vi "configure.vi"(8 "error in (no error)":errorcluster, 11 "lv-build-default in":refnum<class "lv-builder.lvclass">) -> (0 "error out":errorcluster, 3 "lv-build-default out":refnum<class "lv-builder.lvclass">)   [LabVIEW 2015, in "lv-builder.lvlib" / "lv-builder.lvclass"]
uses:
  lv-builder.lvclass
  lv-builder.lvclass/lv-builder.ctl
  private/_controls/command_configuration.ctl
  lv-builder.lvlib
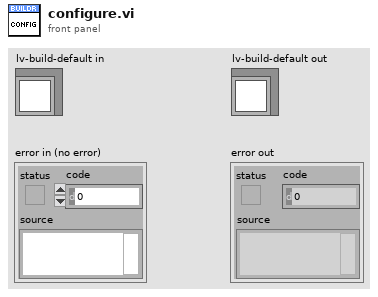
[diagram p1: front panel]
types:
  T1 = typedef "lv-builder.lvlib/command_configuration.ctl" = enum16{"<config_command>", "read_config", "write_config", "<null>"}
  T2 = typedef "lv-builder.lvlib/configuration.ctl" = cluster{"lvlibp_directory":string, "zip_directory":string, "lvlib_directory":string, "update_version_vi":string, "installer_post_file":string, "lvlib_post_action":u16, "installer_post_action":u16, "application_post_action":u16, "zip_post_action":u16}
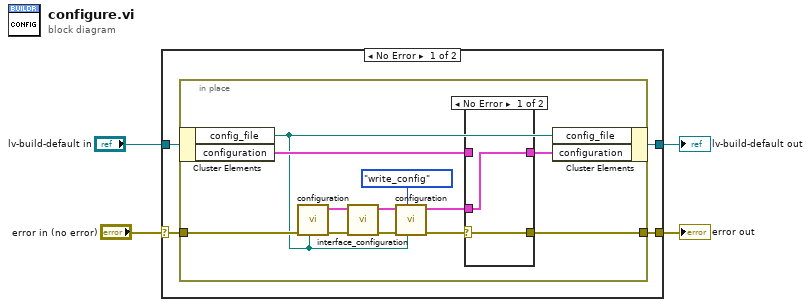
[diagram p0: block diagram]
diagram:
  n1 = case shown="No Error" "error in (no error)" {
    selector: "error in (no error)" -> [w8 w26]
    tunnel: "lv-build-default in" -> [w6 w25]
    tunnel: [w7 w26] -> w2
    tunnel: [w5 w25] -> w1
    frame No Error {
      n2 = in-place {
        in-place-border: w8 -> [w13]
        in-place-border: [w20] -> w7
        n3 = in-place-cluster #1(w6) -> ("config_file"=w9:path, "configuration"=w19:T2)
        n4 = call "configuration.vi"("config_file"=w9, "error in (no error)"=w13) -> ("error out"=w14:errorcluster, "config out"=w17:T2)  [unwired: 8 in]
        n5 = call "interface_configuration.vi"("error in (no error)"=w14, "config in"=w17) -> ("error out"=w15:errorcluster, "config out"=w16:T2)  [unwired: 8 in]
        n6 = call "configuration.vi"("config_file"=w9, "command"=command_configuration."write_config", "error in (no error)"=w15, "config in"=w16) -> ("error out"=w12:errorcluster, "config out"=w11:T2)  [unwired: 6 in]
        n7 = case shown="No Error" w12 {
          selector: w12 -> [w22 w23]
          tunnel: [w22 w23] -> w20
          tunnel: w19 -> [_ w24]
          tunnel: [w21 w24] -> w18
          tunnel: w11 -> [w21 _]
          frame No Error {
          }
          frame Error {
          }
        }
        n8 = in-place-cluster #1("config_file"=w9, "configuration"=w18) -> (w5:refnum<class "lv-builder.lvclass">)
      }
    }
    frame Error {
    }
  }
  "error out" <- w2
  "lv-build-default out" <- w1
